vi "Write Module Name.vi"(8 "error in (no error)":errorcluster, 10 "Module Name":string, 11 "ADAS_IO_Template_MDO in":refnum<class "ADAS_IO_Template_MDO.lvclass">) -> (0 "error out":errorcluster, 3 "ADAS_IO_Template_MDO out":refnum<class "ADAS_IO_Template_MDO.lvclass">)   [LabVIEW 2020, in "ADAS_IO_Template_MDO.lvclass"]
uses:
  ADAS_IO_Template_MDO.lvclass
  ADAS_IO_Template_MDO.lvclass/ADAS_IO_Template_MDO.ctl
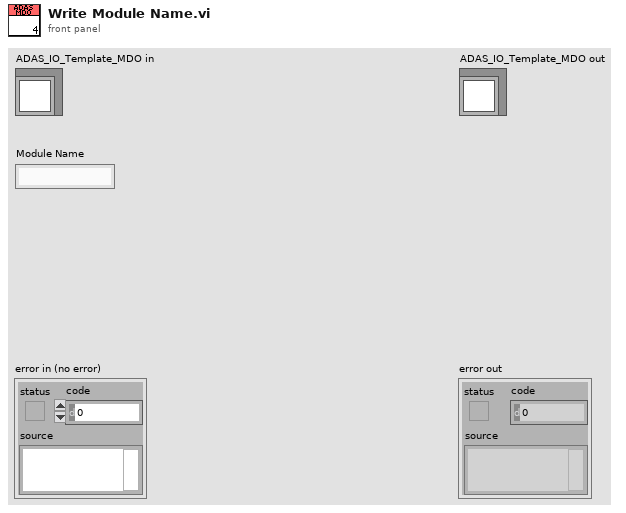
[diagram p1: front panel]
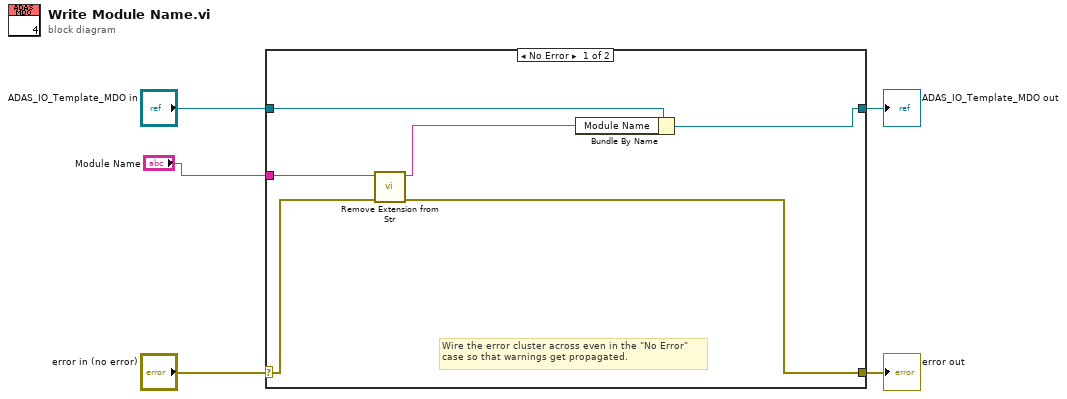
[diagram p0: block diagram]
diagram:
  n1 = case shown="No Error" "error in (no error)" {
    selector: "error in (no error)" -> [w11 w13]
    tunnel: [w10 w13] -> w4
    tunnel: [w6 w12] -> w2
    tunnel: "ADAS_IO_Template_MDO in" -> [w8 w12]
    tunnel: "Module Name" -> [w9 _]
    frame No Error {
      # "Wire the error cluster across even in the \"No Error\"\ncase so that warnings get propagated."
      n2 = call "Remove Extension from Str.vi"("error in (no error)"=w11, "Name"=w9) -> ("error out"=w10:errorcluster, "Name Without Extension"=w7:string)  [unwired: 8 in]
      n3 = Bundle By Name(cluster=w8, "Module Name"=w7) -> (w6:refnum<class "ADAS_IO_Template_MDO.lvclass">)
    }
    frame Error {
    }
  }
  "error out" <- w4
  "ADAS_IO_Template_MDO out" <- w2
